vi "Testbench.vi"() -> ()   [LabVIEW 2015]
uses:
  Interface/Configuration.ctl
  <vilib>/FPGAPlugInAG/sbRIO-9607/niLvFpga_Open_sbRIO-9607.vi
  <vilib>/rvi/interface/common/dynamic/niFpgaDynamicAddResources.vi
  <vilib>/Utility/error.llb/Error Cluster From Error Code.vi
  <vilib>/rvi/errors/niLvFpgaAdjustHostInterfaceError.vi
  <vilib>/FPGAPlugInAG/Dynamic/niLvFpga_Close_Dynamic.vi
  <vilib>/rvi/interface/nirviOpenFPGA/nirviOpenFPGA.xnode
  FPGA Bitfiles/ScaleAndLimit_FPGATarget_BasicFPGATest_5eEjrSJq-IM.lvbitx
  BasicFPGATest.vi
  <vilib>/rvi/interface/nirviReadWriteControl/nirviReadWriteControl.xnode
  <vilib>/rvi/interface/nirviCloseFPGA/nirviCloseFPGA.xnode
  Interface/ScaleAndLimitInterface.lvlib
  NiFpgaLv.dll
  <vilib>/rvi/interface/Simulation/niFpgaSimulationCallBeginRW.vi
panel:
  out "Limits":string
  out "UnscaledAI":i16[](array[numeric])
  in  "DummyAI15":i16
  in  "stop":bool
  out "ScaledAI":sgl[](array[numeric])
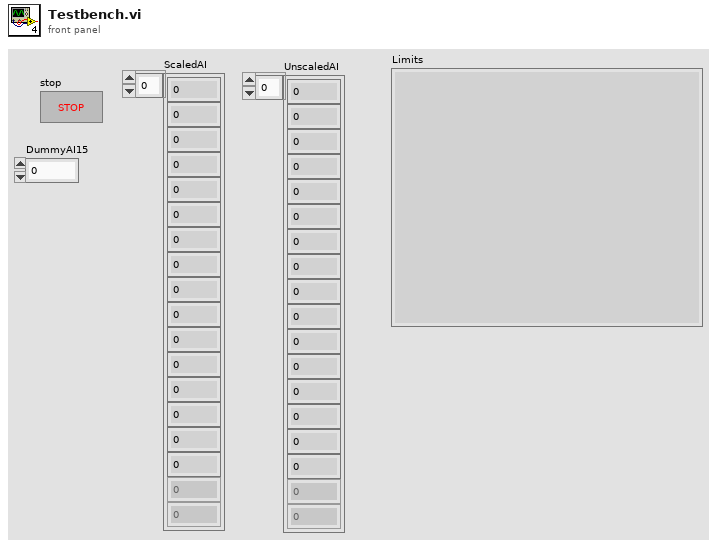
[diagram p1: front panel]
types:
  T1 = typedef "ScaleAndLimitInterface.lvlib/Configuration.ctl" = cluster{"Name":string, "M":dbl, "B":i16, "HighLimit":dbl, "LowLimit":dbl, "LimitsEnabled":bool}
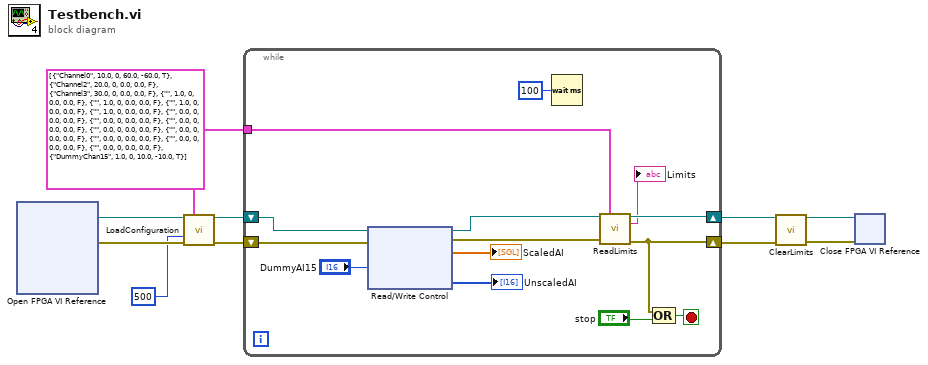
[diagram p0: block diagram]
diagram:
  w6 = T1[] [{"Name"="Channel0", "M"=10.0, "B"=0, "HighLimit"=60.0, "LowLimit"=-60.0, "LimitsEnabled"=TRUE}, {"Name"="Channel2", "M"=20.0, "B"=0, "HighLimit"=0.0, "LowLimit"=0.0, "LimitsEnabled"=FALSE}, {"Name"="Channel3", "M"=30.0, "B"=0, "HighLimit"=0.0, "LowLimit"=0.0, "LimitsEnabled"=FALSE}, {"Name"="", "M"=1.0, "B"=0, "HighLimit"=0.0, "LowLimit"=0.0, "LimitsEnabled"=FALSE}, {"Name"="", "M"=1.0, "B"=0, "HighLimit"=0.0, "LowLimit"=0.0, "LimitsEnabled"=FALSE}, {"Name"="", "M"=1.0, "B"=0, "HighLimit"=0.0, "LowLimit"=0.0, "LimitsEnabled"=FALSE}, {"Name"="", "M"=1.0, "B"=0, "HighLimit"=0.0, "LowLimit"=0.0, "LimitsEnabled"=FALSE}, {"Name"="", "M"=0.0, "B"=0, "HighLimit"=0.0, "LowLimit"=0.0, "LimitsEnabled"=FALSE}, {"Name"="", "M"=0.0, "B"=0, "HighLimit"=0.0, "LowLimit"=0.0, "LimitsEnabled"=FALSE}, {"Name"="", "M"=0.0, "B"=0, "HighLimit"=0.0, "LowLimit"=0.0, "LimitsEnabled"=FALSE}, {"Name"="", "M"=0.0, "B"=0, "HighLimit"=0.0, "LowLimit"=0.0, "LimitsEnabled"=FALSE}, {"Name"="", "M"=0.0, "B"=0, "HighLimit"=0.0, "LowLimit"=0.0, "LimitsEnabled"=FALSE}, {"Name"="", "M"=0.0, "B"=0, "HighLimit"=0.0, "LowLimit"=0.0, "LimitsEnabled"=FALSE}, {"Name"="", "M"=0.0, "B"=0, "HighLimit"=0.0, "LowLimit"=0.0, "LimitsEnabled"=FALSE}, {"Name"="", "M"=0.0, "B"=0, "HighLimit"=0.0, "LowLimit"=0.0, "LimitsEnabled"=FALSE}, {"Name"="DummyChan15", "M"=1.0, "B"=0, "HighLimit"=10.0, "LowLimit"=-10.0, "LimitsEnabled"=TRUE}] ("Configuration")
  n1 = xnode "Open FPGA VI Reference"() -> ("FPGA VI Reference Out"=w5:refnum<k20>, "error out"=w10:errorcluster)  [unwired: 2 in]
  n2 = call "LoadConfiguration.vi"("FPGA Interface in"=w5, "Configuration"=w6, "Timeout (ms)"=500, "error in (no error)"=w10) -> ("FPGA Interface out"=w8:refnum<k20>, "error out"=w7:errorcluster)  [unwired: 10 in]
  n3 = while {
    shift-right: [w15] -> w4
    shift-left: w8 -> [w23]
    shift-right: [w12] -> w2
    shift-left: w7 -> [w24]
    tunnel: w6 -> [w16]
    stop <- w13 stop-if-true
    n4 = xnode "Read/Write Control"("FPGA VI Reference In"=w23, "error in"=w24, "DummyAI15"="DummyAI15") -> ("FPGA VI Reference Out"=w17:refnum<k20>, "error out"=w18:errorcluster, "ScaledAI"=→"ScaledAI":sgl[], "UnscaledAI"=→"UnscaledAI":i16[])
    n5 = Wait (ms)(milliseconds to wait=u32 100) -> ()  [unwired: 1 out]
    n6 = call "ReadLimits.vi"("FPGA Interface in"=w17, "Configuration"=w16, "error in (no error)"=w18) -> ("FPGA Interface out"=w15:refnum<k20>, "Limits"=→"Limits":string, "error out"=w12:errorcluster)  [unwired: 10 in]
    n7 = Compound Arithmetic op=OR(w12, "stop") -> (w13:bool)
  }
  n8 = call "ClearLimits.vi"("FPGA Interface in"=w4, "error in (no error)"=w2) -> ("FPGA Interface out"=w1:refnum<k20>, "error out"=w3:errorcluster)  [unwired: 12 in]
  n9 = xnode "Close FPGA VI Reference"("FPGA VI Reference In"=w1, "error in"=w3) -> ()  [unwired: 1 out]
